vi "VideoCapture_bak.vi"(0 "Output Directory":path=path "C:/Users/dpl/OneDrive - Aberystwyth University/Documents/LabVIEW Data/VideoTest", 1 "SaveFile":string, 3 "error in (no error)":errorcluster, 4 "Path to FFMPEG":path=path "C:/Users/dpl/Downloads/ffmpeg-master-latest-win64-gpl/ffmpeg-master-latest-win64-gpl/bin/ffmpeg.exe", 5 "Duration (s)":dbl=1.0 min=0.0 max=100.0, 6 "Video Camera":string) -> (10 "error out":errorcluster)   [LabVIEW 2024]
doc: "Calls FFMPEG to capture and record a video clip.\nVideo clip is stored in sub-directory VIDEOS from Output directory\n\nFilename derived from Cycle count and nominal temperature (TNOM)\nVideo stampedwith timecode, cycle count and nominal temperature"
panel:
  in  "TNom":dbl
  in  "Cycle":i32
  in  "SaveType":enum16{"WMV", "MP4"}(ring)
  out "return code":i32
  out "command string":string
  out "standard error":string
  out "standard output":string
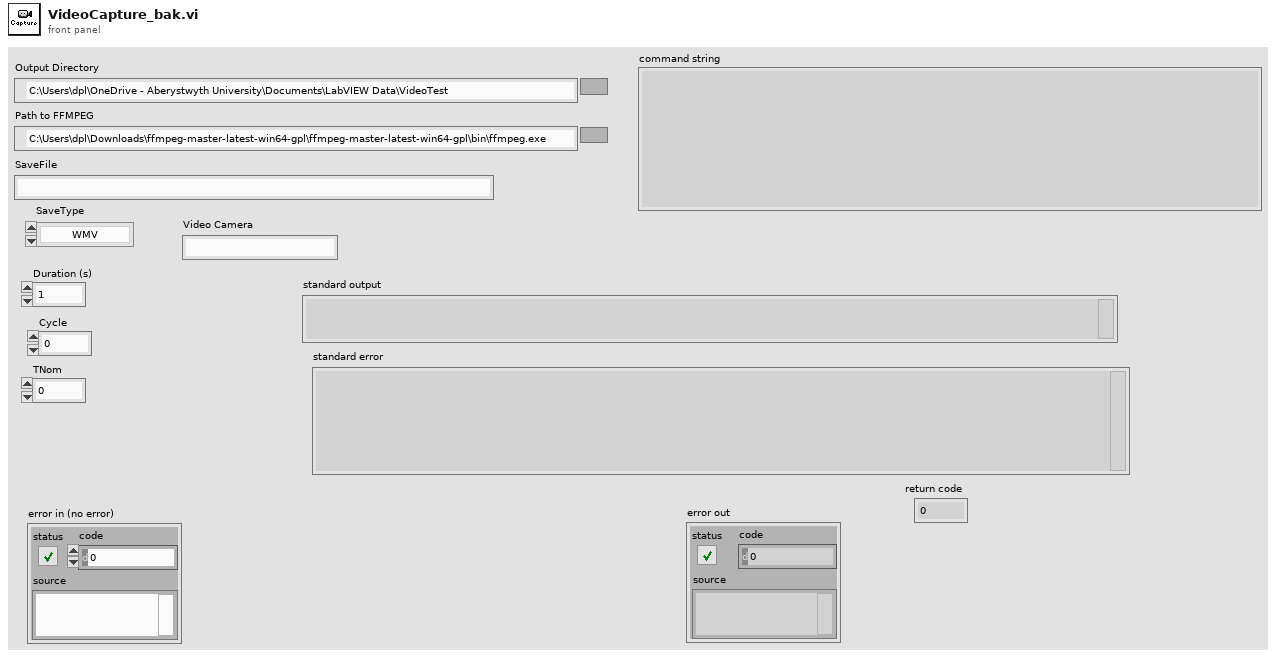
[diagram p1: front panel]
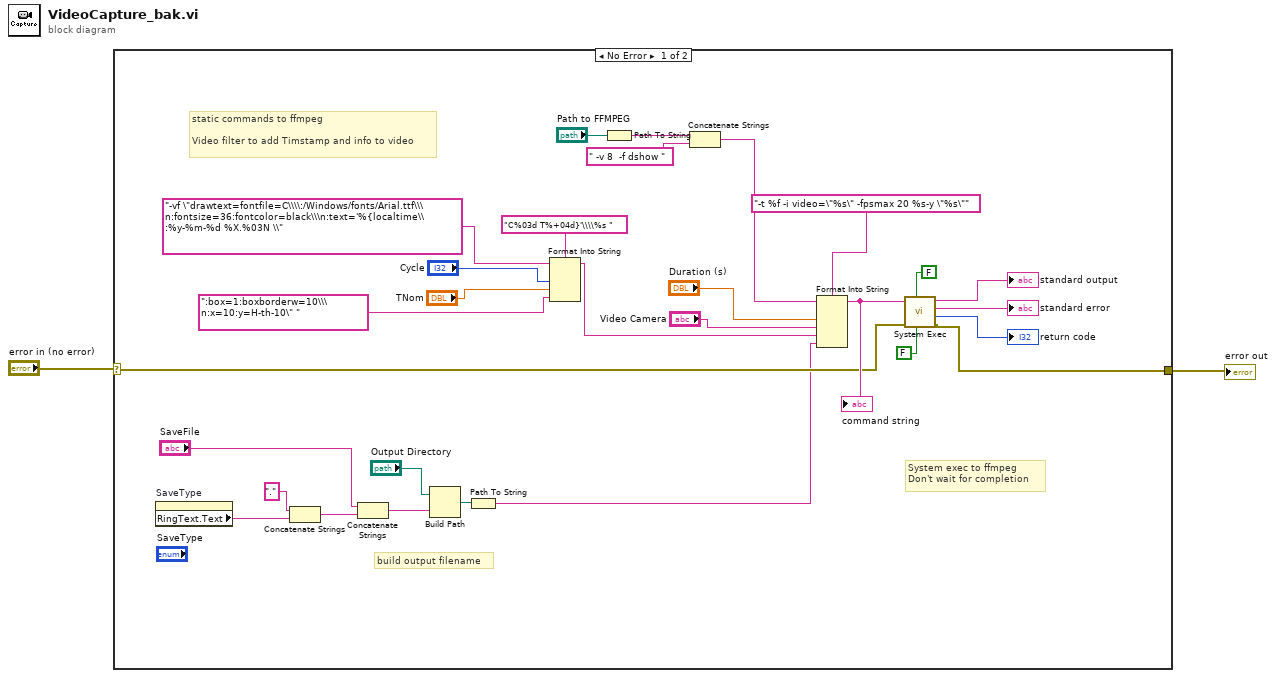
[diagram p0: block diagram]
diagram:
  n1 = case shown="No Error" "error in (no error)" {
    selector: "error in (no error)" -> [w16 w32]
    tunnel: [w17 w32] -> w1
    frame No Error {
      # "build output filename"
      # "System exec to ffmpeg\nDon't wait for completion"
      # "static commands to ffmpeg\n\nVideo filter to add Timstamp and info to video"
      n2 = property on="SaveType" class="Enum (strict)"() -> ("RingText.Text"=w15:string)  [unwired: 2 in, 2 out]
      n3 = Concatenate Strings("." ("string"), w15) -> (w14:string)
      n4 = Concatenate Strings("SaveFile", w14) -> (w19:string)
      n5 = Build Path(base path="Output Directory", name or relative path=w19) -> (appended path=w28:path)
      n6 = Path To String(path=w28) -> (string=w3:string)
      n7 = Format Into String(format string="C%03d T%+04d}'\\\\%s ", initial string="-vf \"drawtext=fontfile=C\\\\:/Windows/fonts/Arial.ttf\\\n:fontsize=36:fontcolor=black\\\n:text='%{localtime\\:%y-%m-%d %X.%03N \\", "Cycle", "TNom", ":box=1:boxborderw=10\\\n:x=10:y=H-th-10\" ") -> (resulting string=w5:string)  [unwired: 1 in, 1 out]
      n8 = Path To String(path="Path to FFMPEG") -> (string=w23:string)
      n9 = Concatenate Strings(w23, " -v 8  -f dshow " ("string")) -> (w12:string)
      n10 = Format Into String(format string="-t %f -i video=\"%s\" -fpsmax 20 %s-y \"%s\"", initial string=w12, "Duration (s)", "Video Camera", w5, w3) -> (resulting string=w21:string)  [unwired: 1 in, 1 out]
      "command string" <- w21
      n11 = call <vilib>:"System Exec.vi"("run minimized? (F)"=FALSE, "wait until completion? (T)"=FALSE, "error in (no error)"=w16, "command line"=w21) -> ("error out"=w17:errorcluster, "return code"=→"return code":i32, "standard error"=→"standard error":string, "standard output"=→"standard output":string)  [unwired: 4 in]
    }
    frame Error {
    }
  }
  "error out" <- w1
